vi "Do This.vi"(8 "error in (no error)":errorcluster, 10 "Status Events":refnum<class "Status Events.lvclass">, 11 "LabVIEW Build in":refnum<class "LabVIEW Build.lvclass">) -> (0 "error out":errorcluster, 3 "LabVIEW Build out":refnum<class "LabVIEW Build.lvclass">)   [LabVIEW 2014, in "LabVIEW Build.lvclass"]
uses:
  LabVIEW Build.lvclass
  Classes/Status Events/Status Events.lvclass
  Classes/Job/Job.lvclass/Job.ctl
  LabVIEW Build.lvclass/LabVIEW Build.ctl
  <vilib>/Utility/error.llb/DialogType.ctl
  <vilib>/AppBuilder/AB_API_Simple/Build (path).vi
  <vilib>/AppBuilder/AB_API_Simple/NI_App_Builder_API.lvlib
  Classes/Job/Job.lvclass
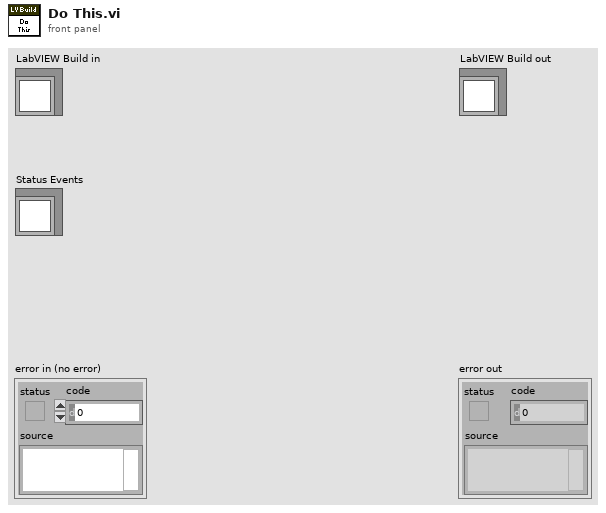
[diagram p1: front panel]
types:
  T1 = typedef "DialogType.ctl" = u16
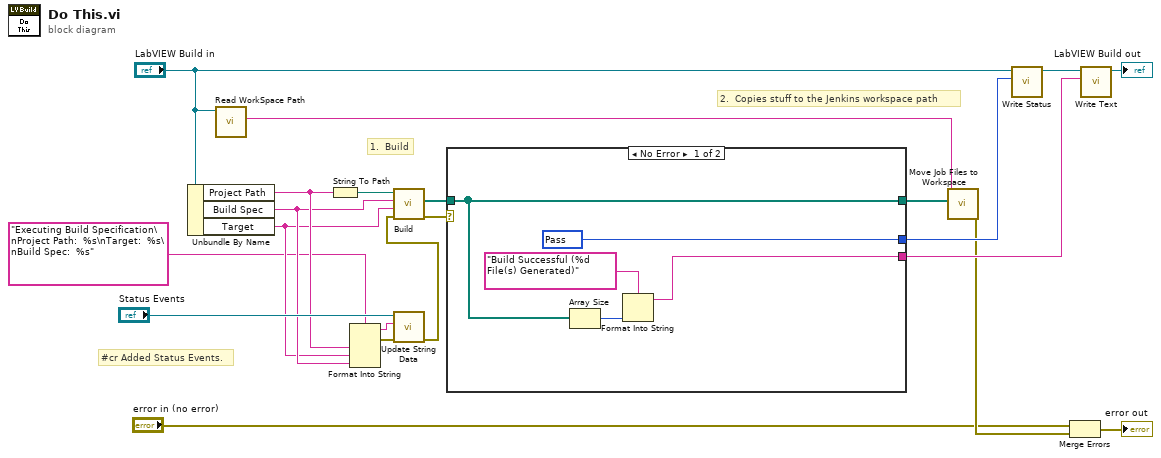
[diagram p0: block diagram]
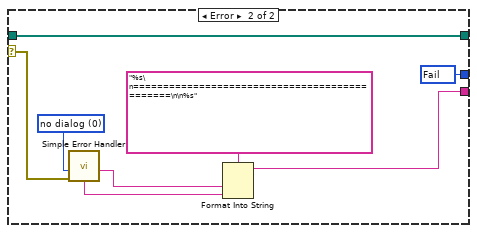
[diagram p2: hidden frame]
diagram:
  # "#cr Added Status Events."
  # "2.  Copies stuff to the Jenkins workspace path"
  # "1.  Build"
  n1 = Unbundle By Name("LabVIEW Build in") -> ("Project Path"=w5:string, "Build Spec"=w4:string, "Target"=w3:string)
  n2 = call "Read WorkSpace Path.vi"("Job in"="LabVIEW Build in") -> ("WorkSpace Path"=w19:string)  [unwired: 8 in, 2 out]
  n3 = String To Path(string=w5) -> (path=w20:path)
  n4 = Format Into String(format string="Executing Build Specification\nProject Path:  %s\nTarget:  %s\nBuild Spec:  %s", w5, w3, w4) -> (resulting string=w7:string, error out=w6:errorcluster)  [unwired: 2 in]
  n5 = call "Update String Data.vi"("error in (no error)"=w6, "String Data"=w7, "Status Updater in"="Status Events") -> ("error out"=w2:errorcluster)  [unwired: 7 in, 1 out]
  n6 = call-poly <vilib>:"Build.vi"("error in (no error)"=w2, "Name of target (My Computer)"=w3, "Name of build specification (if empty: build all)"=w4, "Path to project"=w20) -> ("error out"=w21:errorcluster, "Generated files"=w18:path[])  [unwired: 6 in]
  n7 = case shown="No Error" w21 {
    selector: w21 -> [_ w33]
    tunnel: [w26 w34] -> w16
    tunnel: [w24 w28] -> w15
    tunnel: w18 -> [w22 w27]
    tunnel: [w22 w27] -> w17
    frame No Error {
      w26 = u16 200 items=["Abort"=503, "Fail"=500, "Pass"=200] ("Status")
      n8 = Array Size(array=w22) -> (size(s)=w23:i32)
      n9 = Format Into String(format string="Build Successful (%d File(s) Generated)" ("Text"), w23) -> (resulting string=w24:string)  [unwired: 2 in, 1 out]
    }
    frame Error {
      w32 = T1 0 items=["no dialog", "OK message", "continue or stop message", "OK message + warnings", "continue/stop + warnings"] ("type of dialog (OK msg:1)")
      w34 = u16 500 items=["Abort"=503, "Fail"=500, "Pass"=200] ("Status")
      n10 = call <vilib>:"Simple Error Handler.vi"("type of dialog (OK msg:1)"=w32, "error in (no error)"=w33) -> ("source out"=w30:string, "message"=w29:string)  [unwired: 3 in, 3 out]
      n11 = Format Into String(format string="%s\n==============================================\n\n%s", w30, w29) -> (resulting string=w28:string)  [unwired: 2 in, 1 out]
    }
  }
  n12 = call "Move Job Files to Workspace.vi"("Generated Files"=w17, "Workspace Path"=w19) -> ("error out"=w11:errorcluster)  [unwired: 9 in]
  n13 = call "Write Status.vi"("Status"=w16, "Job in"="LabVIEW Build in") -> ("Job out"=w13:refnum<class "LabVIEW Build.lvclass">)  [unwired: 8 in, 1 out]
  n14 = Merge Errors("error in (no error)", w11) -> (→"error out":errorcluster)
  n15 = call "Write Text.vi"("Text"=w15, "Job in"=w13) -> ("Job out"=→"LabVIEW Build out":refnum<class "LabVIEW Build.lvclass">)  [unwired: 8 in, 1 out]
